vi "Periodic Tasks.vi"(8 "error in":errorcluster) -> ()   [LabVIEW 2016]
doc: "This VI runs in parallel to other tasks. It can contain as many user-defined periodic loops as you need. These can carry out PID or other sorts of timed response."
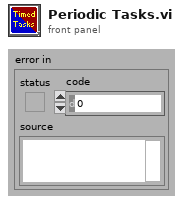
[diagram p1: front panel]
types:
  T1 = typedef "WPI_JoystickDevRef.ctl" = cluster{"Device":T2}
  T2 = typedef "WPI_JoystickDeviceEnum.ctl" = enum16{"USB 0", "USB 1", "USB 2", "USB 3", "USB 4", "USB 5"}
  T3 = typedef "WPI_MotorControlDeviceRef.ctl" = cluster{"DeviceStatus":errorcluster, "Type":T4, "PWM":cluster{"PWM Channel":T5, "DeadBand":T6}, "CAN":cluster{"Device Number":u8, "SetOutput VI Ref":variant, "GetOutput VI Ref":variant, "Enable VI Ref":variant, "Disable VI Ref":variant, "Data":variant}, "Invert":bool}
  T4 = typedef "WPI_MotorControlType.ctl" = enum16{"PWM", "CAN"}
  T5 = typedef "FPGA_DIOPWMChannel.ctl" = enum8{"PWM 0", "PWM 1", "PWM 2", "PWM 3", "PWM 4", "PWM 5", "PWM 6", "PWM 7", "PWM 8", "PWM 9", "PWM MXP 0", "PWM MXP 1", "PWM MXP 2", "PWM MXP 3", "PWM MXP 4", "PWM MXP 5", "PWM MXP 6", "PWM MXP 7", "PWM MXP 8", "PWM MXP 9", "Invalid"}
  T6 = typedef "WPI_PWMDeadband.ctl" = cluster{"Name":string, "maxPositivePwm":i32, "minPositivePwm":i32, "centerPwm":i32, "maxNegativePwm":i32, "minNegativePwm":i32, "angularRange":u16}
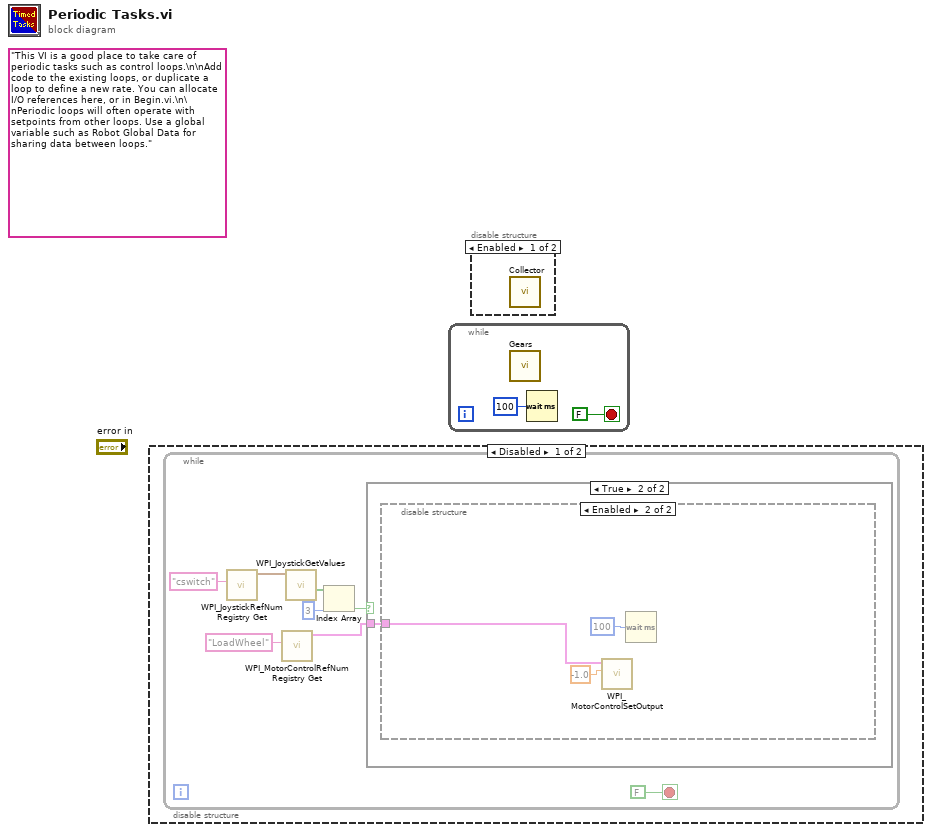
[diagram p0: block diagram]
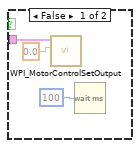
[diagram p2: hidden frame]
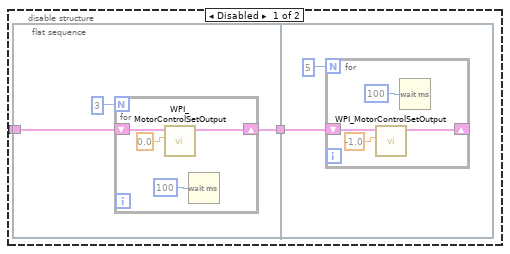
[diagram p3: hidden frame]
diagram:
  (unwired) "This VI is a good place to take care of periodic tasks such as control loops.\n\nAdd code to the existing loops, or duplicate a loop to define a new rate. You can allocate I/O references here, or in Begin.vi.\n\nPeriodic loops will often operate with setpoints from other loops. Use a global variable such as Robot Global Data for sharing data between loops."
  n1 = disable-structure shown="Disabled" {
    frame Disabled {
      n2 = while {
        stop <- FALSE stop-if-true
        n3 = call <vilib>:"WPI_JoystickRefNum Registry Get.vi"("refnum name"="cswitch") -> ("JoystickDevRef"=w6:T1)  [unwired: 9 in, 1 out]
        n4 = call <vilib>:"WPI_MotorControlRefNum Registry Get.vi"("refnum name"="LoadWheel") -> ("MotorControlDevRef"=w1:T3)  [unwired: 9 in, 1 out]
        n5 = call <vilib>:"WPI_JoystickGetValues.vi"("JoystickDevRef"=w6) -> ("Buttons"=w5:bool[])  [unwired: 6 in, 4 out]
        n6 = Index Array(array=w5, index=3) -> (element=w3:bool)
        n7 = case shown="True" w3 {
          tunnel: w1 -> [w9 w12]
          frame False {
            n8 = call <vilib>:"WPI_MotorControlSetOutput.vi"("Output"=0.0, "MotorControlDevRef"=w9) -> ()  [unwired: 7 in, 3 out]
            n9 = Wait (ms)(milliseconds to wait=u32 100) -> ()  [unwired: 1 out]
          }
          frame True {
            n10 = disable-structure shown="Enabled" {
              disable-tunnel: w12 -> [w13 w28]
              frame Disabled {
                n11 = flat-sequence {
                  tunnel: [w17] -> w14
                  tunnel: w13 -> [w16]
                  tunnel: w14 -> [w23]
                  frame #0 {
                    n12 = for {
                      N: 3 -> [_]
                      shift-right: [w21] -> w17
                      shift-left: w16 -> [w20]
                      n13 = call <vilib>:"WPI_MotorControlSetOutput.vi"("Output"=0.0, "MotorControlDevRef"=w20) -> ("MotorControlDevRef"=w21:T3)  [unwired: 7 in, 2 out]
                      n14 = Wait (ms)(milliseconds to wait=u32 100) -> ()  [unwired: 1 out]
                    }
                  }
                  frame #1 {
                    n15 = for {
                      N: 5 -> [_]
                      shift-right: [w27] -> _
                      shift-left: w23 -> [w26]
                      n16 = call <vilib>:"WPI_MotorControlSetOutput.vi"("Output"=-1.0, "MotorControlDevRef"=w26) -> ("MotorControlDevRef"=w27:T3)  [unwired: 7 in, 2 out]
                      n17 = Wait (ms)(milliseconds to wait=u32 100) -> ()  [unwired: 1 out]
                    }
                  }
                }
              }
              frame Enabled {
                n18 = call <vilib>:"WPI_MotorControlSetOutput.vi"("Output"=-1.0, "MotorControlDevRef"=w28) -> ()  [unwired: 7 in, 3 out]
                n19 = Wait (ms)(milliseconds to wait=u32 100) -> ()  [unwired: 1 out]
              }
            }
          }
        }
      }
    }
    frame Enabled {
    }
  }
  n20 = while {
    stop <- FALSE stop-if-true
    n21 = call "Gears.vi"() -> ()  [unwired: 12 in]
    n22 = Wait (ms)(milliseconds to wait=u32 100) -> ()  [unwired: 1 out]
  }
  n23 = disable-structure shown="Enabled" {
    frame Enabled {
      n24 = call "Collector.vi"() -> ()  [unwired: 12 in]
    }
    frame Disabled {
    }
  }
